vi "iterative_segments_to_centerline.vi"(2 "Endpoints":i32[](array[numeric]), 3 "Segment Sequence Cluster Arrays":cluster{i32[]}[](array[cluster])) -> (0 "Timed Out":bool, 1 "Best Centerline 1D":i32[](array[numeric]))   [LabVIEW 2019]
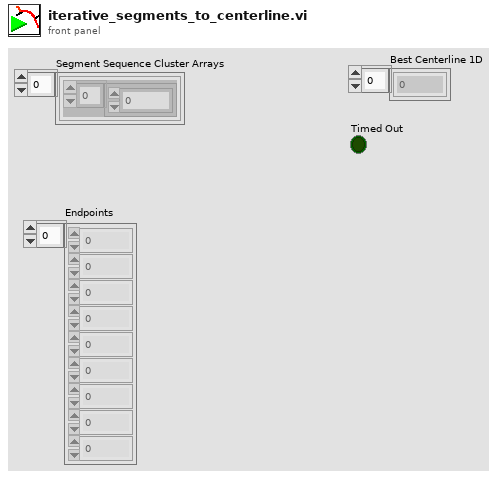
[diagram p1: front panel]
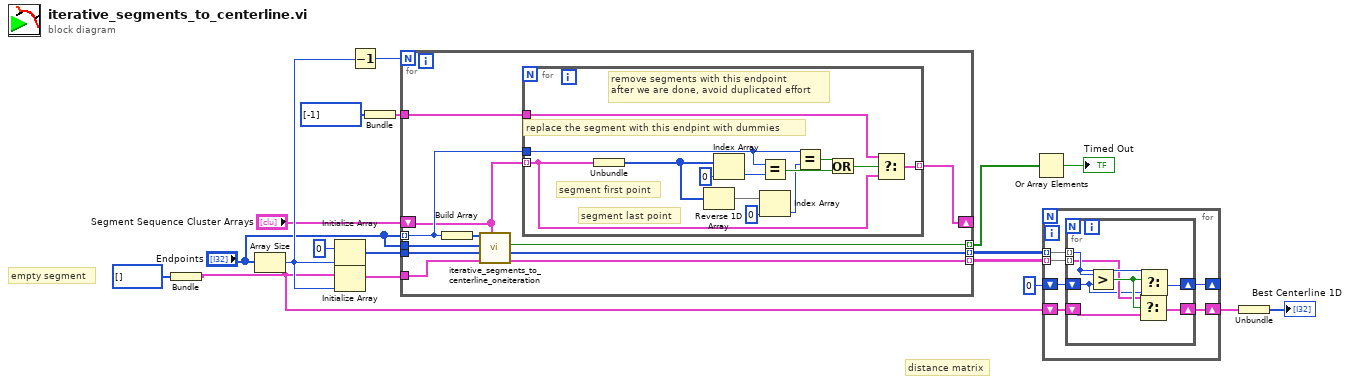
[diagram p0: block diagram]
diagram:
  # "empty segment"
  # "distance matrix"
  n1 = Bundle("Segment Sequence"=i32[] []) -> (w1:cluster{"Segment Sequence":i32[]})  [unwired: 1 in]
  n2 = Array Size(array="Endpoints") -> (size(s)=w14:i32)
  n3 = Initialize Array(0 ("element"), w14) -> (w17:i32[])
  n4 = Initialize Array(w1, w14) -> (w16:cluster{"Segment Sequence":i32[]}[])
  n5 = Decrement(x=w14) -> (x-1=w15:i32)
  n6 = Bundle("Segment Sequence"=i32[] [-1]) -> (w3:cluster{"Segment Sequence":i32[]})  [unwired: 1 in]
  n7 = for {
    N: w15 -> [_]
    tunnel: w17 -> [w29]
    tunnel: "Endpoints" -> [w24] mode=indexing
    tunnel: w16 -> [w28]
    tunnel: [w27] -> w13 mode=indexing
    tunnel: [w26] -> w12 mode=indexing
    tunnel: "Endpoints" -> [w23]
    tunnel: [w22] -> w7 mode=indexing
    shift-right: [w19] -> _
    shift-left: "Segment Sequence Cluster Arrays" -> [w21]
    tunnel: w3 -> [w20]
    n8 = Build Array(w24) -> (w25:i32[])
    n9 = call "iterative_segments_to_centerline_oneiteration.vi"("Segment Sequence Cluster Arrays"=w21, "Potential Centerlines In"=w28, "Potential Centerline Distances In"=w29, "Endpoints"=w23, "Concatenated Segments"=w25) -> ("Potential Centerlines Out"=w26:cluster{i32[]}[], "Potential Centerline Lengths Out"=w27:i32[], "Timed Out"=w22:bool)  [unwired: 4 in]
    n10 = for {
      tunnel: w21 -> [w32] mode=indexing
      tunnel: w24 -> [w38]
      tunnel: w20 -> [w31]
      tunnel: [w30] -> w19 mode=indexing
      # "remove segments with this endpoint\nafter we are done, avoid duplicated effort"
      # "replace the segment with this endpint with dummies"
      # "segment first point"
      # "segment last point"
      n11 = Unbundle(w32) -> (w39:i32[])
      n12 = Reverse 1D Array(array=w39) -> (reversed array=w40:i32[])
      n13 = Index Array(array=w39, index=0) -> (element=w35:i32)
      n14 = Equal?(x=w38, y=w35) -> (x = y?=w36:bool)
      n15 = Index Array(array=w40, index=0) -> (element=w34:i32)
      n16 = Equal?(x=w38, y=w34) -> (x = y?=w37:bool)
      n17 = Or(x=w37, y=w36) -> (x .or. y?=w33:bool)
      n18 = Select(t=w31, s=w33, f=w32) -> (s? t:f=w30:cluster{"Segment Sequence":i32[]})
    }
  }
  n19 = Or Array Elements(Boolean array=w7) -> (logical OR=→"Timed Out":bool)
  n20 = for {
    tunnel: w13 -> [w48] mode=indexing
    tunnel: w12 -> [w47] mode=indexing
    shift-right: [w44] -> _
    shift-left: 0 -> [w46]
    shift-right: [w43] -> w10
    shift-left: w1 -> [w45]
    n21 = for {
      tunnel: w48 -> [w53] mode=indexing
      tunnel: w47 -> [w51] mode=indexing
      shift-right: [w55] -> w44
      shift-left: w46 -> [w50]
      shift-right: [w54] -> w43
      shift-left: w45 -> [w49]
      n22 = Greater?(x=w53, y=w50) -> (0:w52:bool)
      n23 = Select(t=w51, s=w52, f=w49) -> (s? t:f=w54:cluster{"Segment Sequence":i32[]})
      n24 = Select(t=w53, s=w52, f=w50) -> (s? t:f=w55:i32)
    }
  }
  n25 = Unbundle(w10) -> ("Segment Sequence"=→"Best Centerline 1D":i32[])
